vi "P2.vi"(0 "Image In":T1, 1 "File Path (Image Calibration P2)":path=path "C:/Users/serce/Desktop/Smart Vision System Testbench/Grid Calibration.png", 2 "Template File Path (Locate P2 Hole)":path=path "C:/Users/serce/Desktop/Smart Vision System Testbench/P2/P2 Hole Template.png", 7 "Error In":errorcluster) -> (20 "Image Out":T1, 21 "Number of Matches (Locate P2 Hole)":i32, 22 "Fitted Circle (P2 Hole)":T2 {"Average SNR (dB)" format="%.2f"; "Average Strength" format="%.2f"; "Roundness (Real-World)" format="%.2f"; "Radius (Real-World)" format="%.2f"; "Center (Real-World)"."Y" format="%.2f"; "Center (Real-World)"."X" format="%.2f"; "Radius (Pixels)" format="%.2f"; "Center (Pixels)"."Y" format="%.2f"; "Center (Pixels)"."X" format="%.2f"}, 23 "Calibrated Results (P2 Left Edge Angles)":sgl[][](array[numeric]) format="%.2f", 24 "Calibrated Results (P2 Right Edge Angle)":sgl[][](array[numeric]) format="%.2f", 27 "Error Out":errorcluster)   [LabVIEW 2020]
uses:
  <vilib>/vision/Image Controls.llb/IMAQ Image.ctl
  <vilib>/vision/Pattern Matching.llb/IMAQ Curve Parameters.ctl
  <vilib>/vision/Pattern Matching.llb/IMAQ Match Range Setting.ctl
  <vilib>/vision/Pattern Matching.llb/IMAQ Geometric Pattern 2 Advanced Match Options.ctl
  <vilib>/vision/Image Controls.llb/Vision Info Type2.ctl
  <vilib>/vision/Measure.llb/Edge Options.ctl
  <vilib>/vision/Measure.llb/Edge Polarity.ctl
  <vilib>/vision/Measure.llb/Straight Edge Options.ctl
  <vilib>/vision/Measure.llb/Straight Edge Process.ctl
  <vilib>/vision/NI_Vision_Development_Module.lvlib
panel:
  out "Error Out":errorcluster
  out "Image Out":T1
  in  "Error In":errorcluster
  out "Error Out":errorcluster
  in  "Image Dup In":T1
  out "Image Dup Out":T1
  in  "Error In":errorcluster
  in  "Image In":T1
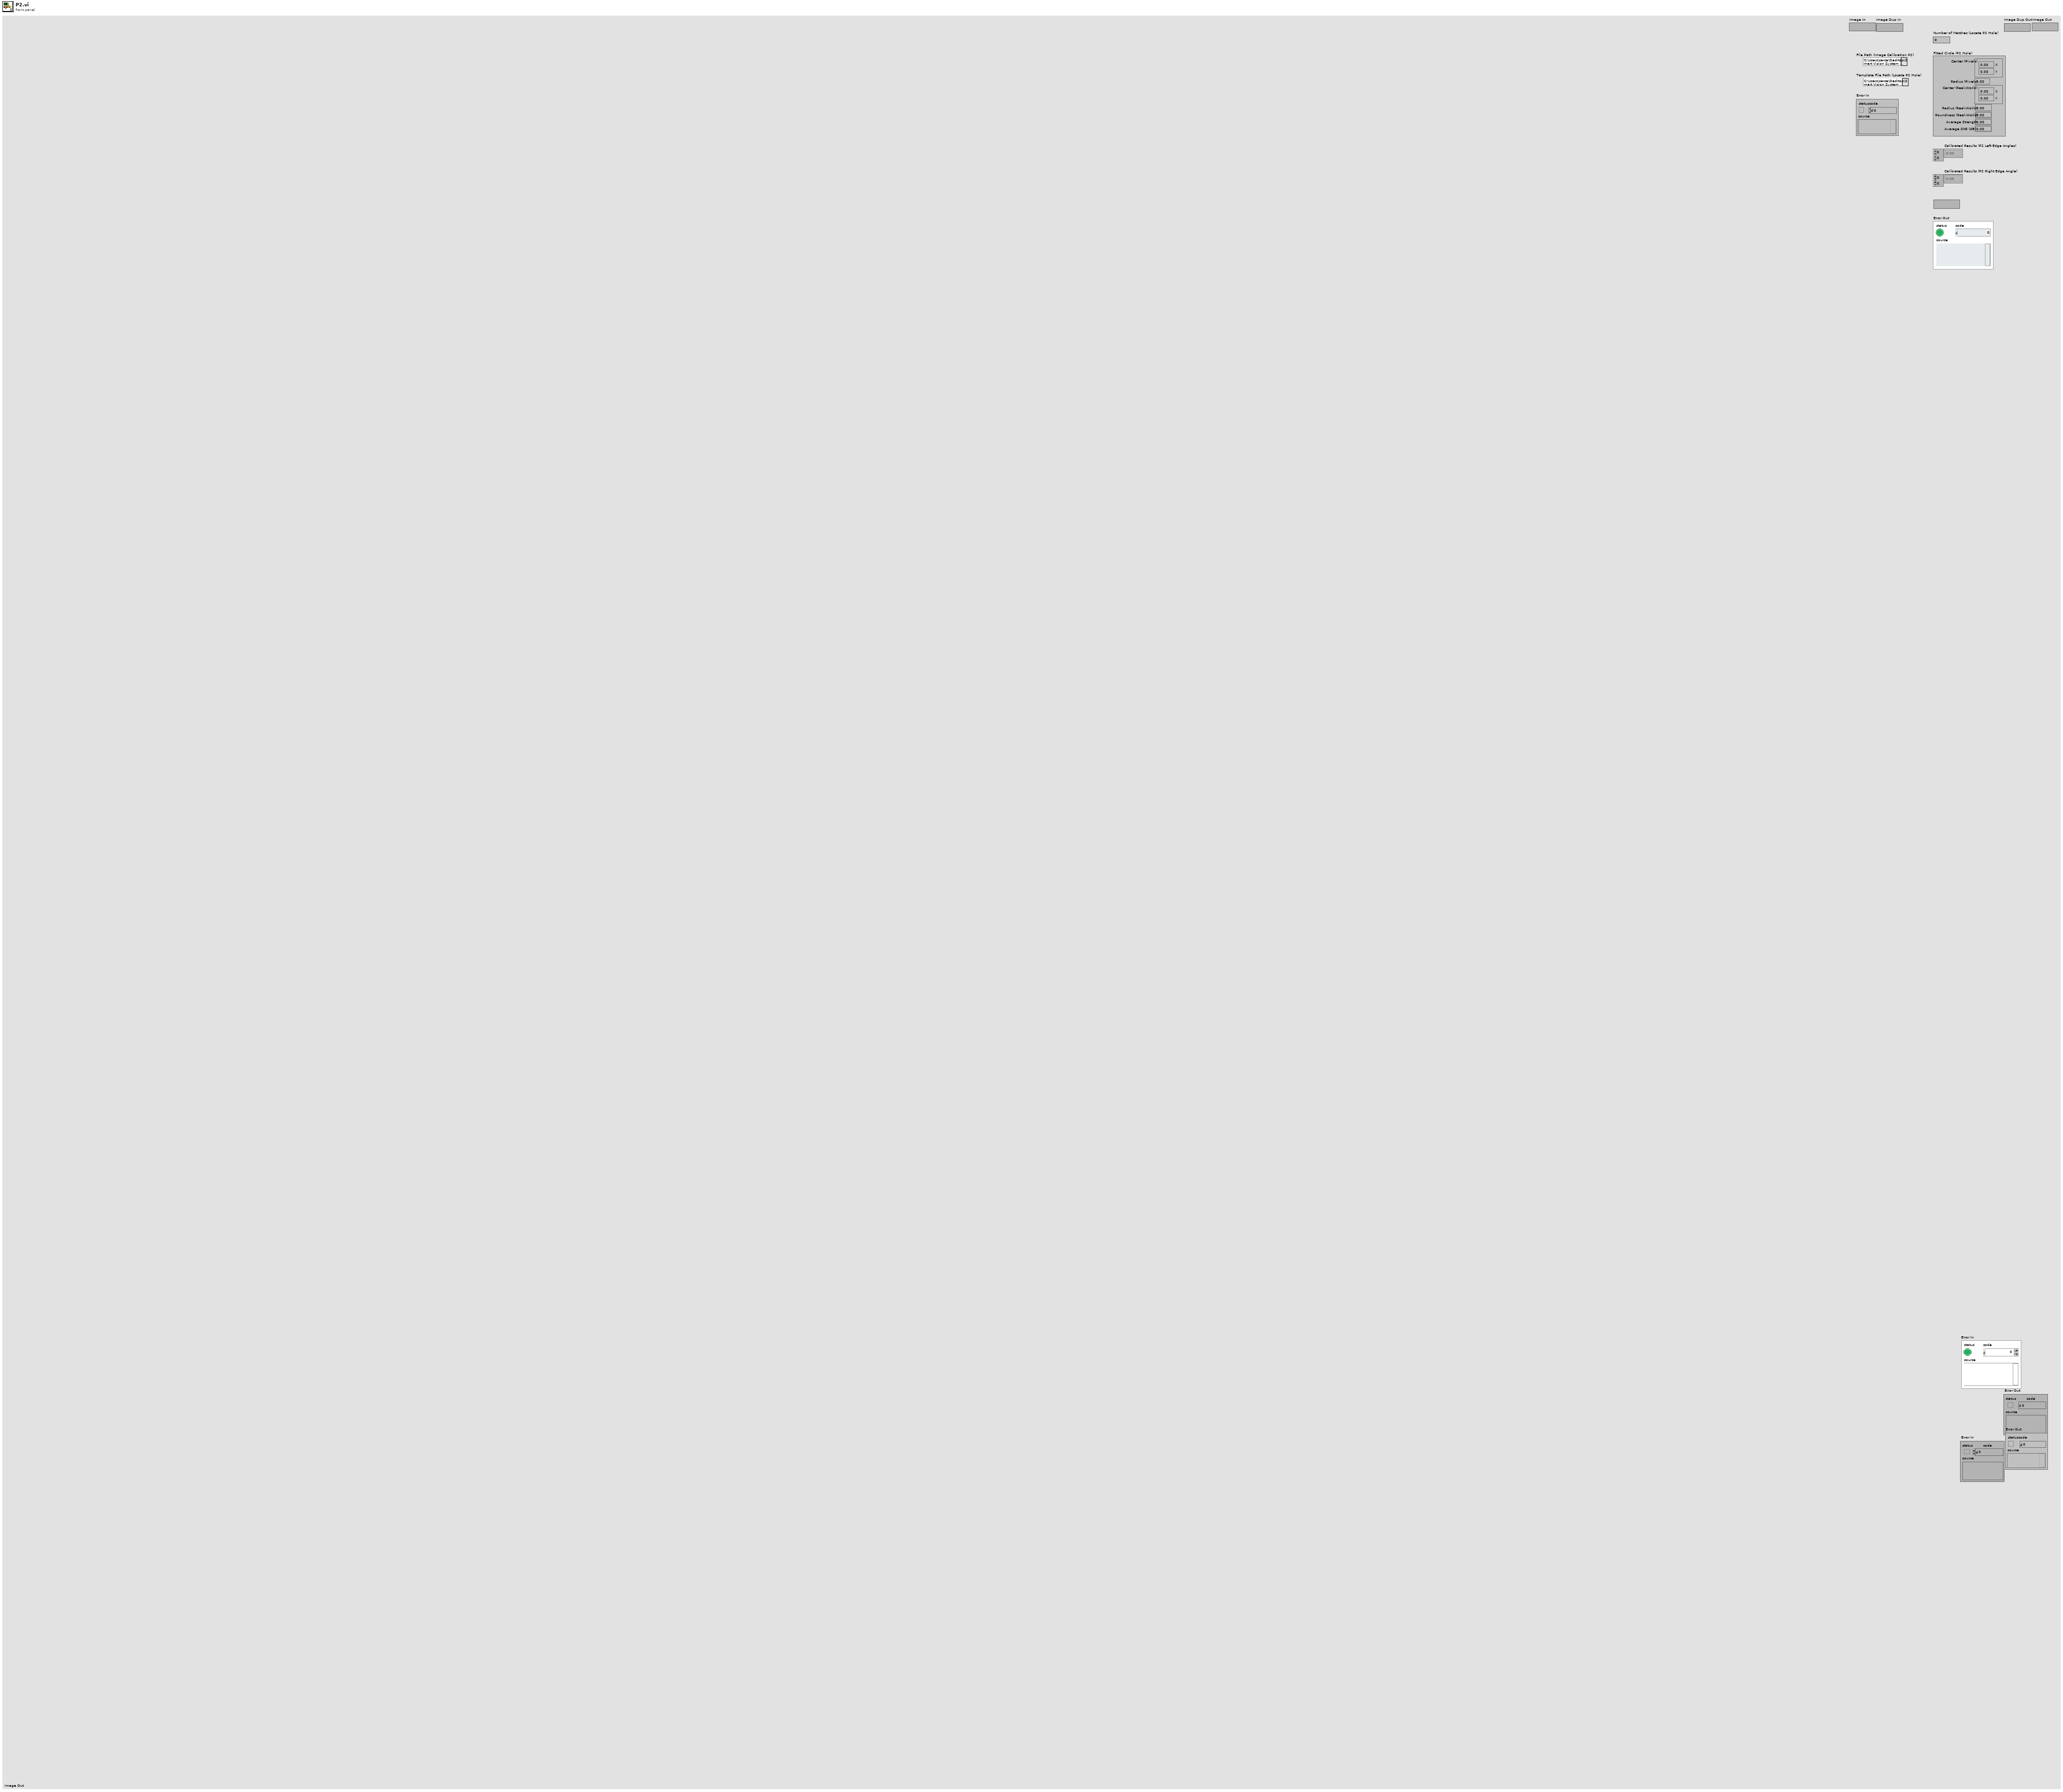
[diagram p1: front panel]
types:
  T1 = typedef "IMAQ Image.ctl" = refnum<image>
  T2 = cluster{"Center (Pixels)":cluster{"X":sgl, "Y":sgl}, "Radius (Pixels)":dbl, "Center (Real-World)":cluster{"X":sgl, "Y":sgl}, "Radius (Real-World)":dbl, "Roundness (Real-World)":dbl, "Average Strength":dbl, "Average SNR (dB)":dbl}
  T3 = cluster{"Feature":u32, "Points IDs":cluster{"GUID":string, "Index":i32}[]}[]
  T4 = typedef "Edge Options.ctl" = cluster{"Edge Polarity":T5, "Kernel Size":u32, "Width":u32, "Minimum Edge Strength":sgl, "Interpolation Type":enum32{"Zero Order", "Bilinear", "Quadratic", "Cubic", "Bilinear Fixed"}, "Data Processing Method":enum32{"Average", "Median"}}
  T5 = typedef "Edge Polarity.ctl" = u32
  T6 = cluster{"Search Direction":u32, "Edge Options":T4, "Show Search Area":bool, "Show Search Lines":bool, "Show Edges Found":bool, "Show Result":bool, "Search Area Color":u32, "Search Lines Color":u32, "Edge Locations Color":u32, "Result Color":u32, "Overlay Group Name":string}
  T7 = typedef "Straight Edge Options.ctl" = cluster{"Number of Lines":i32, "Type":T8, "Min. Score":dbl, "Max. Score":dbl, "Orientation":dbl, "Angle Range":dbl, "Angle Tolerance":dbl, "Step Size":u32, "Min. SNR (db)":dbl, "Min. Points (%)":dbl, "Hough Iterations":i32}
  T8 = typedef "Straight Edge Process.ctl" = enum32{"First Edge Rake", "Best Edge Rake", "Hough Edge Rake", "First Edge Projection", "Best Edge Projection"}
  T9 = cluster{"Global Rectangle":i32[], "Contours":cluster{"ID":enum32{"External", "Internal"}, "Type":u32, "Coordinates":i32[]}[]}
  T10 = cluster{"Origin":cluster{"X":sgl, "Y":sgl}, "Angle (deg)":sgl, "Axis Reference":u32}
  T11 = enum16{"Reset", "Update Coordinate System", "Get Coordinate System"}
  T12 = cluster{"Search  Direction":u32, "Edge Options":T4, "Show Search Area":bool, "Show Search Lines":bool, "Show Edges Found":bool, "Show Result":bool, "Search Area Color":u32, "Search Lines Color":u32, "Edge Locations Color":u32, "Result Color":u32, "Overlay Group Name":string}
  T13 = cluster{"Process":enum16{"Get First Edge", "Get First + Last Edge", "Get All Edges", "Get Best Edge"}, "Step Size":i32, "Max Pixel Radius":i32}
  T14 = cluster{"Origin Pixel":cluster{"X":sgl, "Y":sgl}, "X Axis Pixel":cluster{"X":sgl, "Y":sgl}, "Axis Reference":u32}
  T15 = typedef "Vision Info Type2.ctl" = u32
  T16 = typedef "Simple Grid Descriptor" = cluster{"X Step":sgl, "Y Step":sgl, "Unit":T17}
  T17 = typedef "Image Unit" = enum32{"Undefined", "Angström", "Micrometer", "Millimeter", "Centimeter", "Meter", "Kilometer", "Microinch", "Inch", "Feet", "Nautical miles", "Standard miles", "Steps"}
  T18 = enum16{"Horizontal Motion", "Vertical Motion", "Horizontal and Vertical Motion", "Horizontal, Vertical and Angular Motion"}
  T19 = typedef "IMAQ Curve Parameters.ctl" = cluster{"Extraction Mode":u32, "Edge Threshold":i32, "Edge Filter Size":u32, "Min Length":i32, "Row Search Step Size":i32, "Col Search Step Size":i32, "Max Endpoint Gap":i32, "Closed":bool, "Subpixel":bool}
  T20 = typedef "IMAQ Match Range Setting.ctl" = cluster{"Match Constraints":u32, "Min":dbl, "Max":dbl}
  T21 = typedef "IMAQ Geometric Pattern 2 Advanced Match Options.ctl" = u16
  T22 = cluster{"Curve Parameters":T19, "Match Mode":cluster{"Rotation":bool, "Scale":bool, "Occlusion":bool, "Reserved 1":bool, "Reserved 2":bool, "Reserved 3":bool}, "Range Settings":T20[], "Number of Matches":i32, "Minimum Match Score":sgl, "SubPixel Accuracy":bool, "Adv. Geometric Match Options 2":cluster{"Setup Data Item":T21, "Item Value":dbl}[]}
  T23 = cluster{"Brightness":sgl, "Contrast":sgl, "Gamma":sgl}
  T24 = typedef "IMAQ GM Match Report.ctl" = cluster{"Position":cluster{"x":sgl, "y":sgl}, "Angle":sgl, "Scale":sgl, "Score":sgl, "Bounding Box":cluster{"x":sgl, "y":sgl}[], "Contrast Reversed":bool, "Occlusion %":sgl, "Template Target Curve Score":sgl, "Target Template Curve Score":sgl, "Correlation Score":sgl}
  T25 = typedef "IMAQ Coordinate System" = cluster{"Reference System":cluster{"Origin":cluster{"X":sgl, "Y":sgl}, "Angle (deg)":sgl, "Axis Reference":u32}, "Measurement System":cluster{"Origin":cluster{"X":sgl, "Y":sgl}, "Angle (deg)":sgl, "Axis Reference":u32}}
  T26 = typedef "ROI Descriptor" = cluster{"Global Rectangle":i32[], "Contours":cluster{"ID":enum32{"External", "Internal"}, "Type":u32, "Coordinates":i32[]}[]}
  T27 = cluster{"Point1 (Pixels)":cluster{"X":sgl, "Y":sgl}, "Point2 (Pixels)":cluster{"X":sgl, "Y":sgl}, "Point1 (Real-World)":cluster{"X":sgl, "Y":sgl}, "Point2 (Real-World)":cluster{"X":sgl, "Y":sgl}, "Angle (Pixel)":dbl, "Angle (Real-World)":dbl, "Score":dbl, "Straightness":dbl, "Average SNR (db)":dbl, "Calibration Valid":bool}[]
  T28 = cluster{"Point1 (Pixels)":cluster{"X":sgl, "Y":sgl}, "Point2 (Pixels)":cluster{"X":sgl, "Y":sgl}, "Point1 (Real-World)":cluster{"X":sgl, "Y":sgl}, "Point2 (Real-World)":cluster{"X":sgl, "Y":sgl}, "Angle (Pixel)":dbl, "Angle (Real-World)":dbl, "Score":dbl, "Straightness":dbl, "Average SNR (db)":dbl, "Calibration Valid":bool}
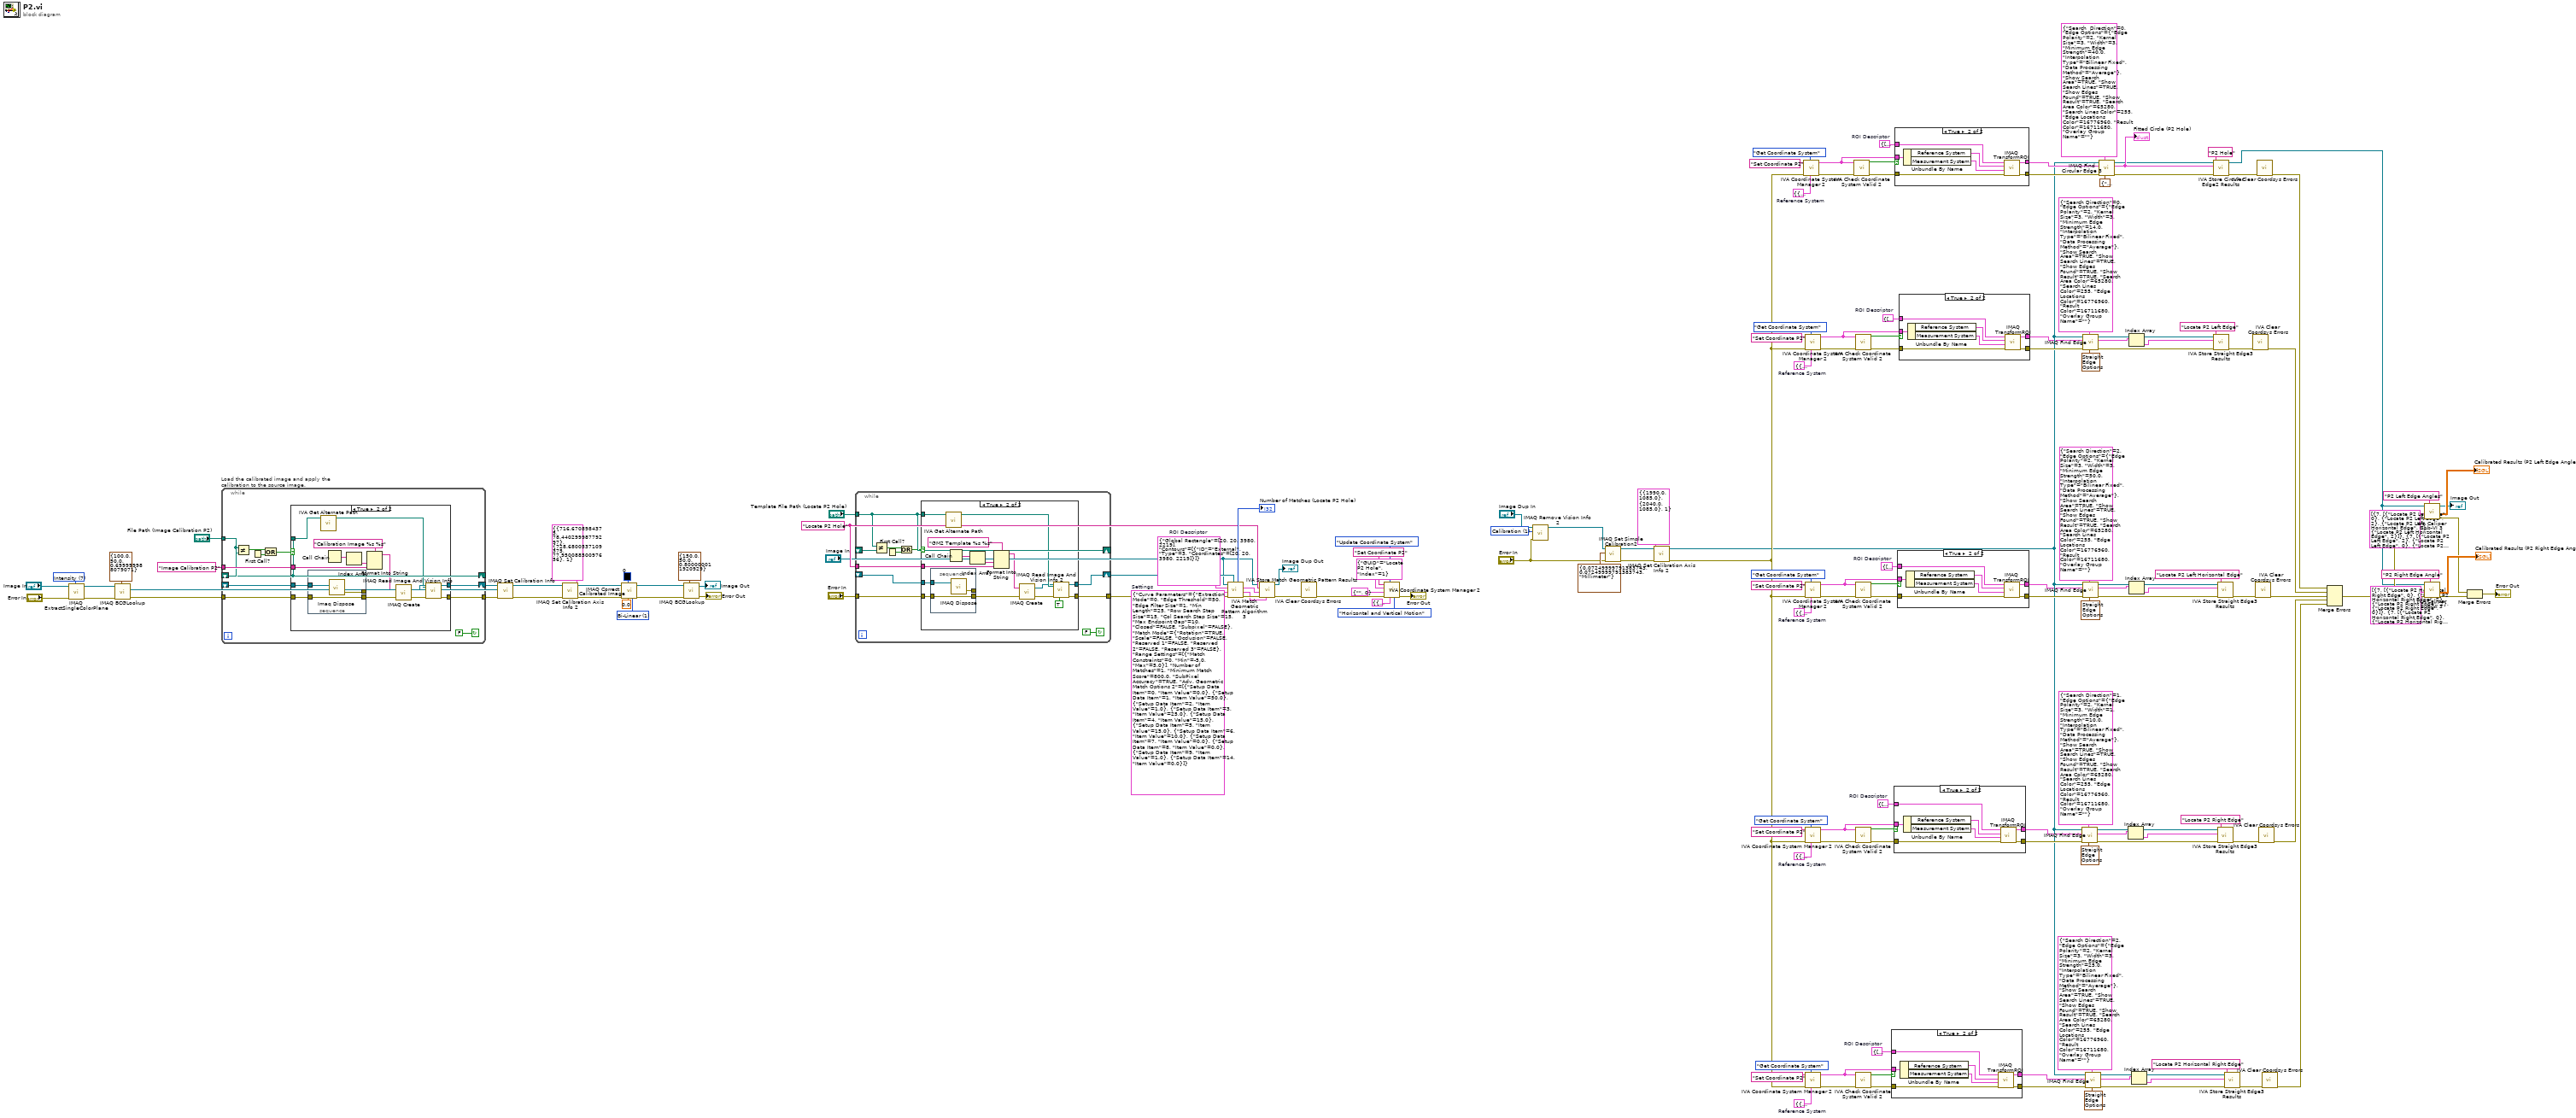
[diagram p0: block diagram]
diagram:
  w47 = T9 {"Global Rectangle"=[2305, 827, 2590, 1102], "Contours"=[{"ID"=enum."External", "Type"=12, "Coordinates"=[2305, 827, 2590, 1102, 0]}]}  # ROI Descriptor
  w48 = T10 {"Origin"={"X"=2091.9243, "Y"=1142.8302}, "Angle (deg)"=0.0, "Axis Reference"=0}  # Reference System
  w66 = T9 {"Global Rectangle"=[2233, 374, 2483, 755], "Contours"=[{"ID"=enum."External", "Type"=12, "Coordinates"=[2233, 374, 2483, 755, 0]}]}  # ROI Descriptor
  w67 = T10 {"Origin"={"X"=2157.2554, "Y"=1094.1909}, "Angle (deg)"=0.0, "Axis Reference"=0}  # Reference System
  w83 = T9 {"Global Rectangle"=[1389, 887, 1708, 1045], "Contours"=[{"ID"=enum."External", "Type"=12, "Coordinates"=[1389, 887, 1708, 1045, 0]}]}  # ROI Descriptor
  w84 = T10 {"Origin"={"X"=2157.2554, "Y"=1094.1909}, "Angle (deg)"=0.0, "Axis Reference"=0}  # Reference System
  w99 = T9 {"Global Rectangle"=[1545, 441, 1957, 867], "Contours"=[{"ID"=enum."External", "Type"=12, "Coordinates"=[1545, 441, 1957, 867, 0]}]}  # ROI Descriptor
  w100 = T10 {"Origin"={"X"=2157.2554, "Y"=1094.1909}, "Angle (deg)"=0.0, "Axis Reference"=0}  # Reference System
  w115 = T9 {"Global Rectangle"=[1957, 954, 2225, 1221], "Contours"=[{"ID"=enum."External", "Type"=7, "Coordinates"=[2090, 1087, 59, 133, 0, 0]}]}  # ROI Descriptor
  w116 = T10 {"Origin"={"X"=2091.9944, "Y"=1085.0201}, "Angle (deg)"=0.0, "Axis Reference"=0}  # Reference System
  w6 = T15 1 items=["Any", "Calibration", "Overlay", "Grayscale Template", "Color Template", "Geometric Template", "Custom Data", "Golden Template", "Geometric Template 2", "Contour Data", "Camera Model"] ("Vision Info")
  w135 = T22 {"Curve Parameters"={"Extraction Mode"=0, "Edge Threshold"=50, "Edge Filter Size"=1, "Min Length"=25, "Row Search Step Size"=15, "Col Search Step Size"=15, "Max Endpoint Gap"=10, "Closed"=FALSE, "Subpixel"=FALSE}, "Match Mode"={"Rotation"=TRUE, "Scale"=FALSE, "Occlusion"=FALSE, "Reserved 1"=FALSE, "Reserved 2"=FALSE, "Reserved 3"=FALSE}, "Range Settings"=[{"Match Constraints"=0, "Min"=-5.0, "Max"=5.0}], "Number of Matches"=1, "Minimum Match Score"=800.0, "SubPixel Accuracy"=TRUE, "Adv. Geometric Match Options 2"=[{"Setup Data Item"=0, "Item Value"=0.0}, {"Setup Data Item"=1, "Item Value"=50.0}, {"Setup Data Item"=2, "Item Value"=1.0}, {"Setup Data Item"=3, "Item Value"=25.0}, {"Setup Data Item"=4, "Item Value"=15.0}, {"Setup Data Item"=5, "Item Value"=15.0}, {"Setup Data Item"=6, "Item Value"=10.0}, {"Setup Data Item"=7, "Item Value"=0.0}, {"Setup Data Item"=8, "Item Value"=0.0}, {"Setup Data Item"=9, "Item Value"=1.0}, {"Setup Data Item"=14, "Item Value"=0.0}]}  # Settings
  w134 = "Locate P2 Hole" ("Step Name")
  w140 = T9 {"Global Rectangle"=[20, 20, 3980, 2219], "Contours"=[{"ID"=enum."External", "Type"=3, "Coordinates"=[20, 20, 3980, 2219]}]}  # ROI Descriptor
  w149 = u32 1 items=["Zero Order", "Bi-Linear", "Quadratic", "Cubic Spline"] ("Interpolation Type")
  w163 = 7 items=["Red", "Green", "Blue", "Hue", "Saturation", "Luminance", "Value", "Intensity"] ("Color Plane")
  n1 = call "IMAQ ExtractSingleColorPlane"("Color Plane"=w163, "error in (no error)"="Error In", "Image Src"="Image In") -> ("error out"=w159:errorcluster, "Image Dst Out"=w160:T1)  [unwired: 1 in, 6 out]
  n2 = call "IMAQ BCGLookup"("Image Src"=w160, "BCG Values"=T23 {"Brightness"=100.0, "Contrast"=50.0, "Gamma"=0.7}, "error in (no error)"=w159) -> ("Image Dst Out"=w153:T1, "error out"=w157:errorcluster)  [unwired: 2 in, 2 out]
  n3 = while "Load the calibrated image and apply the calibration to the source image." {
    shift-right: [w174] -> w155
    shift-left: _ -> [w173]
    tunnel: [w171] -> w154
    tunnel: w157 -> [w170]
    tunnel: "File Path (Image Calibration P2)" -> [w164]
    tunnel: "Image Calibration P2" ("Step Name") -> [w169]
    shift-right: [w164] -> _
    shift-left: _ -> [w165]
    stop <- FALSE continue-if-true
    n4 = Not Equal?(x=w164, y=w165) -> (x != y?=w167:bool)
    n5 = First Call?() -> (First Call?: T/F=w168:bool)
    n6 = Or(x=w167, y=w168) -> (x .or. y?=w166:bool)
    n7 = case shown="True" w166 {
      tunnel: [w176 w188] -> w174
      tunnel: w173 -> [w176 w180]
      tunnel: [w175 w185] -> w171
      tunnel: w170 -> [w175 w181]
      tunnel: w164 -> [_ w178]
      tunnel: w169 -> [_ w182]
      frame False {
      }
      frame True {
        n8 = stacked-sequence {
          tunnel: w181 -> [w192]
          tunnel: w180 -> [w193]
          tunnel: [w192] -> w179
          tunnel: [w191] -> _
          frame #0 {
            n9 = call "Imaq Dispose"("Image"=w193) -> ("error out"=w191:errorcluster)  [unwired: 2 in, 3 out]
          }
        }
        n10 = call <vilib>:"IVA Get Alternate Path.vi"("Path In"=w178) -> ("Path Out"=w177:path)  [unwired: 10 out]
        n11 = Call Chain() -> (call chain=w184:string[])
        n12 = Index Array(array=w184) -> (element=w183:string)  [unwired: 1 in]
        n13 = Format Into String(format string="Calibration Image %s %s" ("Image Name"), w183, w182) -> (resulting string=w190:string)  [unwired: 2 in, 1 out]
        n14 = call "IMAQ Create"("Image Name"=w190, "error in (no error)"=w179) -> ("New Image"=w187:T1, "error out"=w186:errorcluster)  [unwired: 2 in, 1 out]
        n15 = call "IMAQ Read Image And Vision Info"("File Path"=w177, "error in (no error)"=w186, "Image"=w187) -> ("error out"=w185:errorcluster, "Image Out"=w188:T1)  [unwired: 1 in, 6 out]
      }
    }
  }
  n16 = call "IMAQ Set Calibration Info"("error in (no error)"=w154, "Image Dst"=w153, "Image Src"=w155) -> ("error out"=w151:errorcluster, "Calibrated Image"=w15:T1)  [unwired: 1 in, 6 out]
  n17 = call-poly "IMAQ Set Calibration Axis Info 2"("error in (no error)"=w151, "Calibration Axis Info"=T14 {"Origin Pixel"={"X"=716.6709, "Y"=78.4403}, "X Axis Pixel"={"X"=728.68005, "Y"=77.95009}, "Axis Reference"=1}, "Calibration Template Image In"=w15) -> ("error out"=w147:errorcluster, "Calibration Template Image Out"=w148:T1)  [unwired: 7 out]
  n18 = call "IMAQ Correct Calibrated Image"("Interpolation Type"=w149, "Replace Value"=sgl 0.0, "Color Replace Value"=u32 0, "error in (no error)"=w147, "Image Src"=w148) -> ("error out"=w143:errorcluster, "Corrected Image"=w144:T1)  [unwired: 2 in, 3 out]
  n19 = call "IMAQ BCGLookup"("Image Src"=w144, "BCG Values"=T23 {"Brightness"=150.0, "Contrast"=50.0, "Gamma"=0.8}, "error in (no error)"=w143) -> ("Image Dst Out"=→"Image Out":T1, "error out"=→"Error Out":errorcluster)  [unwired: 2 in, 2 out]
  n20 = while {
    shift-right: [w204] -> w132
    shift-left: _ -> [w203]
    tunnel: [w201] -> w133
    tunnel: "Error In" -> [w200]
    tunnel: "Template File Path (Locate P2 Hole)" -> [w197]
    tunnel: w134 -> [w199]
    shift-right: [w197] -> _
    shift-left: _ -> [w198]
    stop <- FALSE continue-if-true
    n21 = Not Equal?(x=w197, y=w198) -> (x != y?=w195:bool)
    n22 = First Call?() -> (First Call?: T/F=w196:bool)
    n23 = Or(x=w195, y=w196) -> (x .or. y?=w194:bool)
    n24 = case shown="True" w194 {
      tunnel: [w206 w208] -> w204
      tunnel: w203 -> [w206 w215]
      tunnel: [w205 w210] -> w201
      tunnel: w200 -> [w205 w216]
      tunnel: w199 -> [_ w217]
      tunnel: w197 -> [_ w214]
      frame False {
      }
      frame True {
        n25 = stacked-sequence {
          tunnel: w216 -> [w224]
          tunnel: w215 -> [w223]
          tunnel: [w224] -> w213
          tunnel: [w222] -> _
          frame #0 {
            n26 = call "IMAQ Dispose"("Image"=w223) -> ("error out"=w222:errorcluster)  [unwired: 2 in, 3 out]
          }
        }
        n27 = call <vilib>:"IVA Get Alternate Path.vi"("Path In"=w214) -> ("Path Out"=w209:path)  [unwired: 10 out]
        n28 = Call Chain() -> (call chain=w219:string[])
        n29 = Index Array(array=w219) -> (element=w218:string)  [unwired: 1 in]
        n30 = Format Into String(format string="GM2 Template %s %s" ("Image Name"), w218, w217) -> (resulting string=w221:string)  [unwired: 2 in, 1 out]
        n31 = call "IMAQ Create"("Image Name"=w221, "error in (no error)"=w213) -> ("New Image"=w207:T1, "error out"=w211:errorcluster)  [unwired: 2 in, 1 out]
        n32 = call "IMAQ Read Image And Vision Info 2"("Use File Path Image Type"=TRUE, "File Path"=w209, "error in (no error)"=w211, "Image"=w207) -> ("error out"=w210:errorcluster, "Image Out"=w208:T1)  [unwired: 5 in, 1 out]
      }
    }
  }
  n33 = call <vilib>:"IVA Match Geometric Pattern Algorithm 3.vi"("Template"=w132, "error in (no error)"=w133, "Settings"=w135, "ROI Descriptor"=w140, "Image"="Image In") -> ("error out"=w139:errorcluster, "Calibrated Matches"=w137:T24[], "Matches"=w138:T24[], "Number of Matches"=→"Number of Matches (Locate P2 Hole)":i32)  [unwired: 3 out]
  n34 = call <vilib>:"IVA Store Match Geometric Pattern Results.vi"("Calibrated Matches"=w137, "error in (no error)"=w139, "Matches"=w138, "Step Name"=w134, "Image in"="Image In") -> ("error out"=w131:errorcluster, "Image dup"=→"Image Dup Out":T1)  [unwired: 5 out]
  n35 = call <vilib>:"IVA Clear Coordsys Errors.vi"("error in (no error)"=w131) -> ("error out"=w124:errorcluster)  [unwired: 10 in]
  n36 = call <vilib>:"IVA Coordinate System Manager 2.vi"("Mode"=T18."Horizontal and Vertical Motion", "Reference System"=T10 {"Origin"={"X"=2091.9944, "Y"=1085.0201}, "Angle (deg)"=0.0, "Axis Reference"=0}, "Function"=T11."Update Coordinate System", "error in (no error)"=w124, "Angle ID"=cluster{"GUID":string, "Index":i32} {"GUID"="", "Index"=0}, "Origin ID"=cluster{"GUID":string, "Index":i32} {"GUID"="Locate P2 Hole", "Index"=1}, "Coordinate System Name"="Set Coordinate P2") -> ("error out"=→"Error Out":errorcluster)  [unwired: 4 out]
  n37 = call "IMAQ Remove Vision Info 2"("error in (no error)"="Error In", "Vision Info"=w6, "Image"="Image Dup In") -> ("Image Out"=w122:T1)  [unwired: 8 out]
  n38 = call "IMAQ Set Simple Calibration2"("error in (no error)"="Error In", "Pixel Distances"=T16 {"X Step"=0.0725, "Y Step"=0.0725, "Unit"=enum."Millimeter"} ("Grid Descriptor"), "Image"=w122) -> ("error out"=w120:errorcluster, "Calibration Template Image"=w121:T1)  [unwired: 2 in, 5 out]
  n39 = call-poly "IMAQ Set Calibration Axis Info 2"("error in (no error)"=w120, "Calibration Axis Info"=T14 {"Origin Pixel"={"X"=1990.0, "Y"=1085.0}, "X Axis Pixel"={"X"=2040.0, "Y"=1085.0}, "Axis Reference"=1}, "Calibration Template Image In"=w121) -> ("error out"=w49:errorcluster, "Calibration Template Image Out"=w42:T1)  [unwired: 7 out]
  n40 = call <vilib>:"IVA Coordinate System Manager 2.vi"("Reference System"=w116, "Function"=T11."Get Coordinate System", "error in (no error)"=w49, "Coordinate System Name"="Set Coordinate P2") -> ("error out"=w112:errorcluster, "Coordinate System Out"=w114:T25)  [unwired: 3 in, 3 out]
  n41 = call <vilib>:"IVA Coordinate System Manager 2.vi"("Reference System"=w100, "Function"=T11."Get Coordinate System", "error in (no error)"=w49, "Coordinate System Name"="Set Coordinate P2") -> ("error out"=w97:errorcluster, "Coordinate System Out"=w5:T25)  [unwired: 3 in, 3 out]
  n42 = call <vilib>:"IVA Coordinate System Manager 2.vi"("Reference System"=w84, "Function"=T11."Get Coordinate System", "error in (no error)"=w49, "Coordinate System Name"="Set Coordinate P2") -> ("error out"=w80:errorcluster, "Coordinate System Out"=w82:T25)  [unwired: 3 in, 3 out]
  n43 = call <vilib>:"IVA Coordinate System Manager 2.vi"("Reference System"=w67, "Function"=T11."Get Coordinate System", "error in (no error)"=w49, "Coordinate System Name"="Set Coordinate P2") -> ("error out"=w63:errorcluster, "Coordinate System Out"=w65:T25)  [unwired: 3 in, 3 out]
  n44 = call <vilib>:"IVA Coordinate System Manager 2.vi"("Reference System"=w48, "Function"=T11."Get Coordinate System", "error in (no error)"=w49, "Coordinate System Name"="Set Coordinate P2") -> ("error out"=w44:errorcluster, "Coordinate System Out"=w46:T25)  [unwired: 3 in, 3 out]
  n45 = call <vilib>:"IVA Check Coordinate System Valid 2.vi"("error in (no error)"=w112, "Coordinate System"=w114) -> ("error out"=w111:errorcluster, "Valid?"=w113:bool)  [unwired: 8 out]
  n46 = call <vilib>:"IVA Check Coordinate System Valid 2.vi"("error in (no error)"=w97, "Coordinate System"=w5) -> ("error out"=w96:errorcluster, "Valid?"=w98:bool)  [unwired: 8 out]
  n47 = call <vilib>:"IVA Check Coordinate System Valid 2.vi"("error in (no error)"=w80, "Coordinate System"=w82) -> ("error out"=w79:errorcluster, "Valid?"=w81:bool)  [unwired: 8 out]
  n48 = call <vilib>:"IVA Check Coordinate System Valid 2.vi"("error in (no error)"=w63, "Coordinate System"=w65) -> ("error out"=w62:errorcluster, "Valid?"=w64:bool)  [unwired: 8 out]
  n49 = call <vilib>:"IVA Check Coordinate System Valid 2.vi"("error in (no error)"=w44, "Coordinate System"=w46) -> ("error out"=w43:errorcluster, "Valid?"=w45:bool)  [unwired: 8 out]
  n50 = case shown="True" w45 {
    tunnel: w47 -> [w226 w233]
    tunnel: [w226 w230] -> w41
    tunnel: [w225 w229] -> w39
    tunnel: w46 -> [_ w228]
    tunnel: w43 -> [w225 w227]
    frame False {
    }
    frame True {
      n51 = Unbundle By Name(w228) -> ("Reference System"=w232:T10, "Measurement System"=w231:T10)
      n52 = call "IMAQ TransformROI"("error in (no error)"=w227, "New Reference"=w231, "Base Reference"=w232, "ROI Descriptor"=w233) -> ("error out"=w229:errorcluster, "ROI Descriptor out"=w230:T26)  [unwired: 6 out]
    }
  }
  n53 = case shown="True" w64 {
    tunnel: w66 -> [w235 w242]
    tunnel: [w235 w239] -> w61
    tunnel: [w234 w238] -> w59
    tunnel: w65 -> [_ w237]
    tunnel: w62 -> [w234 w236]
    frame False {
    }
    frame True {
      n54 = Unbundle By Name(w237) -> ("Reference System"=w241:T10, "Measurement System"=w240:T10)
      n55 = call "IMAQ TransformROI"("error in (no error)"=w236, "New Reference"=w240, "Base Reference"=w241, "ROI Descriptor"=w242) -> ("error out"=w238:errorcluster, "ROI Descriptor out"=w239:T26)  [unwired: 6 out]
    }
  }
  n56 = case shown="True" w113 {
    tunnel: w115 -> [w244 w251]
    tunnel: [w244 w248] -> w109
    tunnel: [w243 w247] -> w108
    tunnel: w114 -> [_ w246]
    tunnel: w111 -> [w243 w245]
    frame False {
    }
    frame True {
      n57 = Unbundle By Name(w246) -> ("Reference System"=w250:T10, "Measurement System"=w249:T10)
      n58 = call "IMAQ TransformROI"("error in (no error)"=w245, "New Reference"=w249, "Base Reference"=w250, "ROI Descriptor"=w251) -> ("error out"=w247:errorcluster, "ROI Descriptor out"=w248:T26)  [unwired: 6 out]
    }
  }
  n59 = case shown="True" w81 {
    tunnel: w83 -> [w253 w260]
    tunnel: [w253 w257] -> w4
    tunnel: [w252 w256] -> w77
    tunnel: w82 -> [_ w255]
    tunnel: w79 -> [w252 w254]
    frame False {
    }
    frame True {
      n60 = Unbundle By Name(w255) -> ("Reference System"=w259:T10, "Measurement System"=w258:T10)
      n61 = call "IMAQ TransformROI"("error in (no error)"=w254, "New Reference"=w258, "Base Reference"=w259, "ROI Descriptor"=w260) -> ("error out"=w256:errorcluster, "ROI Descriptor out"=w257:T26)  [unwired: 6 out]
    }
  }
  n62 = case shown="True" w98 {
    tunnel: w99 -> [w262 w269]
    tunnel: [w262 w266] -> w3
    tunnel: [w261 w265] -> w94
    tunnel: w5 -> [_ w264]
    tunnel: w96 -> [w261 w263]
    frame False {
    }
    frame True {
      n63 = Unbundle By Name(w264) -> ("Reference System"=w268:T10, "Measurement System"=w267:T10)
      n64 = call "IMAQ TransformROI"("error in (no error)"=w263, "New Reference"=w267, "Base Reference"=w268, "ROI Descriptor"=w269) -> ("error out"=w265:errorcluster, "ROI Descriptor out"=w266:T26)  [unwired: 6 out]
    }
  }
  n65 = call "IMAQ Find Edge"("Line Fit Options"=T7 {"Number of Lines"=1, "Type"=enum."First Edge Rake", "Min. Score"=10.0, "Max. Score"=1000.0, "Orientation"=0.0, "Angle Range"=45.0, "Angle Tolerance"=1.0, "Step Size"=38, "Min. SNR (db)"=0.0, "Min. Points (%)"=25.0, "Hough Iterations"=5} ("Fit Options"), "Options"=T6 {"Search Direction"=1, "Edge Options"={"Edge Polarity"=2, "Kernel Size"=3, "Width"=1, "Minimum Edge Strength"=10.0, "Interpolation Type"=enum."Bilinear Fixed", "Data Processing Method"=enum."Average"}, "Show Search Area"=TRUE, "Show Search Lines"=TRUE, "Show Edges Found"=TRUE, "Show Result"=TRUE, "Search Area Color"=65280, "Search Lines Color"=255, "Edge Locations Color"=16776960, "Result Color"=16711680, "Overlay Group Name"=""}, "error in (no error)"=w59, "ROI Descriptor"=w61, "Image"=w42) -> ("error out"=w54:errorcluster, "Straight Edges"=w53:T27, "Image Out"=w55:T1)  [unwired: 1 in, 3 out]
  n66 = call "IMAQ Find Edge"("Line Fit Options"=T7 {"Number of Lines"=1, "Type"=enum."First Edge Rake", "Min. Score"=10.0, "Max. Score"=1000.0, "Orientation"=0.0, "Angle Range"=45.0, "Angle Tolerance"=1.0, "Step Size"=43, "Min. SNR (db)"=0.0, "Min. Points (%)"=25.0, "Hough Iterations"=5} ("Fit Options"), "Options"=T6 {"Search Direction"=0, "Edge Options"={"Edge Polarity"=2, "Kernel Size"=3, "Width"=3, "Minimum Edge Strength"=14.0, "Interpolation Type"=enum."Bilinear Fixed", "Data Processing Method"=enum."Average"}, "Show Search Area"=TRUE, "Show Search Lines"=TRUE, "Show Edges Found"=TRUE, "Show Result"=TRUE, "Search Area Color"=65280, "Search Lines Color"=255, "Edge Locations Color"=16776960, "Result Color"=16711680, "Overlay Group Name"=""}, "error in (no error)"=w94, "ROI Descriptor"=w3, "Image"=w42) -> ("error out"=w89:errorcluster, "Straight Edges"=w88:T27, "Image Out"=w90:T1)  [unwired: 1 in, 3 out]
  n67 = call "IMAQ Find Edge"("Line Fit Options"=T7 {"Number of Lines"=1, "Type"=enum."First Edge Rake", "Min. Score"=10.0, "Max. Score"=1000.0, "Orientation"=0.0, "Angle Range"=45.0, "Angle Tolerance"=1.0, "Step Size"=32, "Min. SNR (db)"=0.0, "Min. Points (%)"=25.0, "Hough Iterations"=5} ("Fit Options"), "Options"=T6 {"Search Direction"=2, "Edge Options"={"Edge Polarity"=2, "Kernel Size"=3, "Width"=3, "Minimum Edge Strength"=50.0, "Interpolation Type"=enum."Bilinear Fixed", "Data Processing Method"=enum."Average"}, "Show Search Area"=TRUE, "Show Search Lines"=TRUE, "Show Edges Found"=TRUE, "Show Result"=TRUE, "Search Area Color"=65280, "Search Lines Color"=255, "Edge Locations Color"=16776960, "Result Color"=16711680, "Overlay Group Name"=""}, "error in (no error)"=w77, "ROI Descriptor"=w4, "Image"=w42) -> ("error out"=w72:errorcluster, "Straight Edges"=w71:T27, "Image Out"=w73:T1)  [unwired: 1 in, 3 out]
  n68 = call "IMAQ Find Edge"("Line Fit Options"=T7 {"Number of Lines"=1, "Type"=enum."First Edge Rake", "Min. Score"=10.0, "Max. Score"=1000.0, "Orientation"=0.0, "Angle Range"=45.0, "Angle Tolerance"=1.0, "Step Size"=28, "Min. SNR (db)"=0.0, "Min. Points (%)"=25.0, "Hough Iterations"=5} ("Fit Options"), "Options"=T6 {"Search Direction"=2, "Edge Options"={"Edge Polarity"=2, "Kernel Size"=3, "Width"=3, "Minimum Edge Strength"=25.0, "Interpolation Type"=enum."Bilinear Fixed", "Data Processing Method"=enum."Average"}, "Show Search Area"=TRUE, "Show Search Lines"=TRUE, "Show Edges Found"=TRUE, "Show Result"=TRUE, "Search Area Color"=65280, "Search Lines Color"=255, "Edge Locations Color"=16776960, "Result Color"=16711680, "Overlay Group Name"=""}, "error in (no error)"=w39, "ROI Descriptor"=w41, "Image"=w42) -> ("error out"=w34:errorcluster, "Straight Edges"=w33:T27, "Image Out"=w35:T1)  [unwired: 1 in, 3 out]
  n69 = call "IMAQ Find Circular Edge 3"("Circle Fit Options"=T13 {"Process"=enum."Get Best Edge", "Step Size"=10, "Max Pixel Radius"=3}, "Options"=T12 {"Search  Direction"=0, "Edge Options"={"Edge Polarity"=2, "Kernel Size"=3, "Width"=3, "Minimum Edge Strength"=40.0, "Interpolation Type"=enum."Bilinear Fixed", "Data Processing Method"=enum."Average"}, "Show Search Area"=TRUE, "Show Search Lines"=TRUE, "Show Edges Found"=TRUE, "Show Result"=TRUE, "Search Area Color"=65280, "Search Lines Color"=255, "Edge Locations Color"=16776960, "Result Color"=16711680, "Overlay Group Name"=""}, "error in (no error)"=w108, "ROI Descriptor"=w109, "Image"=w42) -> ("error out"=w2:errorcluster, "Fitted Circle"=w106:T2, "Image Out"=w104:T1)  [unwired: 2 in, 2 out]
  "Fitted Circle (P2 Hole)" <- w106
  n70 = Index Array(array=w53) -> (element=w56:T28)  [unwired: 1 in]
  n71 = Index Array(array=w88) -> (element=w91:T28)  [unwired: 1 in]
  n72 = Index Array(array=w71) -> (element=w74:T28)  [unwired: 1 in]
  n73 = Index Array(array=w33) -> (element=w36:T28)  [unwired: 1 in]
  n74 = call <vilib>:"IVA Store Circular Edge2 Results.vi"("error in (no error)"=w2, "Step Name"="P2 Hole", "Fitted Circle"=w106, "Image in"=w104) -> ("error out"=w103:errorcluster, "Image dup"=w1:T1)  [unwired: 2 in, 4 out]
  n75 = call <vilib>:"IVA Store Straight Edge3 Results.vi"("error in (no error)"=w89, "Step Name"="Locate P2 Left Edge", "Straight Edge"=w91, "Image in"=w90) -> ("error out"=w87:errorcluster)  [unwired: 1 in, 6 out]
  n76 = call <vilib>:"IVA Store Straight Edge3 Results.vi"("error in (no error)"=w72, "Step Name"="Locate P2 Left Horizontal Edge", "Straight Edge"=w74, "Image in"=w73) -> ("error out"=w70:errorcluster)  [unwired: 1 in, 6 out]
  n77 = call <vilib>:"IVA Store Straight Edge3 Results.vi"("error in (no error)"=w54, "Step Name"="Locate P2 Right Edge", "Straight Edge"=w56, "Image in"=w55) -> ("error out"=w52:errorcluster)  [unwired: 1 in, 6 out]
  n78 = call <vilib>:"IVA Store Straight Edge3 Results.vi"("error in (no error)"=w34, "Step Name"="Locate P2 Horizontal Right Edge", "Straight Edge"=w36, "Image in"=w35) -> ("error out"=w32:errorcluster)  [unwired: 1 in, 6 out]
  n79 = call <vilib>:"IVA Clear Coordsys Errors.vi"("error in (no error)"=w87) -> ("error out"=w30:errorcluster)  [unwired: 10 in]
  n80 = call <vilib>:"IVA Clear Coordsys Errors.vi"("error in (no error)"=w70) -> ("error out"=w29:errorcluster)  [unwired: 10 in]
  n81 = call <vilib>:"IVA Clear Coordsys Errors.vi"("error in (no error)"=w103) -> ("error out"=w31:errorcluster)  [unwired: 10 in]
  n82 = call <vilib>:"IVA Clear Coordsys Errors.vi"("error in (no error)"=w52) -> ("error out"=w28:errorcluster)  [unwired: 10 in]
  n83 = call <vilib>:"IVA Clear Coordsys Errors.vi"("error in (no error)"=w32) -> ("error out"=w27:errorcluster)  [unwired: 10 in]
  n84 = Merge Errors(w31, w30, w29, w28, w27) -> (w23:errorcluster)
  n85 = call <vilib>:"IVA Caliper Sub-VI 3.vi"("error in"=w23, "Parameters"=T3 [{"Feature"=7, "Points IDs"=[{"GUID"="Locate P2 Left Edge", "Index"=0}, {"GUID"="Locate P2 Left Edge", "Index"=2}, {"GUID"="Locate P2 Left Horizontal Edge", "Index"=0}, {"GUID"="Locate P2 Left Horizontal Edge", "Index"=2}]}, {"Feature"=7, "Points IDs"=[{"GUID"="Locate P2 Left Edge", "Index"=2}, {"GUID"="Locate P2 Left Edge", "Index"=0}, {"GUID"="Locate P2 Left Horizontal Edge", "Index"=2}, {"GUID"="Locate P2 Left Horizontal Edge", "Index"=0}]}, {"Feature"=7, "Points IDs"=[{"GUID"="Locate P2 Left Edge", "Index"=0}, {"GUID"="Locate P2 Left Edge", "Index"=2}, {"GUID"="Locate P2 Left Horizontal Edge", "Index"=0}, {"GUID"="Locate P2 Left Horizontal Edge", "Index"=2}]}], "Step Name"="P2 Left Edge Angles", "Image In"=w1) -> ("error out"=w17:errorcluster, "Results (Calibrated)"=→"Calibrated Results (P2 Left Edge Angles)":sgl[][], "Image Out"=→"Image Out":T1)  [unwired: 1 in, 4 out]
  n86 = call <vilib>:"IVA Caliper Sub-VI 3.vi"("error in"=w23, "Parameters"=T3 [{"Feature"=7, "Points IDs"=[{"GUID"="Locate P2 Horizontal Right Edge", "Index"=0}, {"GUID"="Locate P2 Horizontal Right Edge", "Index"=2}, {"GUID"="Locate P2 Right Edge", "Index"=2}, {"GUID"="Locate P2 Right Edge", "Index"=0}]}, {"Feature"=7, "Points IDs"=[{"GUID"="Locate P2 Horizontal Right Edge", "Index"=0}, {"GUID"="Locate P2 Horizontal Right Edge", "Index"=2}, {"GUID"="Locate P2 Right Edge", "Index"=2}, {"GUID"="Locate P2 Right Edge", "Index"=0}]}, {"Feature"=7, "Points IDs"=[{"GUID"="Locate P2 Horizontal Right Edge", "Index"=0}, {"GUID"="Locate P2 Horizontal Right Edge", "Index"=2}, {"GUID"="Locate P2 Right Edge", "Index"=2}, {"GUID"="Locate P2 Right Edge", "Index"=0}]}, {"Feature"=7, "Points IDs"=[{"GUID"="Locate P2 Horizontal Right Edge", "Index"=0}, {"GUID"="Locate P2 Horizontal Right Edge", "Index"=2}, {"GUID"="Locate P2 Right Edge", "Index"=2}, {"GUID"="Locate P2 Right Edge", "Index"=0}]}, {"Feature"=7, "Points IDs"=[{"GUID"="Locate P2 Horizontal Right Edge", "Index"=0}, {"GUID"="Locate P2 Horizontal Right Edge", "Index"=2}, {"GUID"="Locate P2 Right Edge", "Index"=2}, {"GUID"="Locate P2 Right Edge", "Index"=0}]}, {"Feature"=7, "Points IDs"=[{"GUID"="Locate P2 Horizontal Right Edge", "Index"=0}, {"GUID"="Locate P2 Horizontal Right Edge", "Index"=2}, {"GUID"="Locate P2 Right Edge", "Index"=2}, {"GUID"="Locate P2 Right Edge", "Index"=0}]}, {"Feature"=7, "Points IDs"=[{"GUID"="Locate P2 Horizontal Right Edge", "Index"=0}, {"GUID"="Locate P2 Horizontal Right Edge", "Index"=2}, {"GUID"="Locate P2 Right Edge", "Index"=2}, {"GUID"="Locate P2 Right Edge", "Index"=0}]}, {"Feature"=7, "Points IDs"=[{"GUID"="Locate P2 Horizontal Right Edge", "Index"=0}, {"GUID"="Locate P2 Horizontal Right Edge", "Index"=2}, {"GUID"="Locate P2 Right Edge", "Index"=2}, {"GUID"="Locate P2 Right Edge", "Index"=0}]}], "Step Name"="P2 Right Edge Angle", "Image In"=w1) -> ("error out"=w16:errorcluster, "Results (Calibrated)"=→"Calibrated Results (P2 Right Edge Angle)":sgl[][])  [unwired: 1 in, 5 out]
  n87 = Merge Errors(w17, w16) -> (→"Error Out":errorcluster)
